vi "Calibration-NormalizeData.vi"(8 "error in (no error)":errorcluster, 11 "Calibration-RunTest in":refnum<class "Calibration-RunTest.lvclass">) -> (0 "error out":errorcluster, 3 "Calibration-RunTest out":refnum<class "Calibration-RunTest.lvclass">)   [LabVIEW 2013, in "Calibration-RunTest.lvclass"]
uses:
  Calibration-RunTest.lvclass
  Calibration-RunTest.lvclass/Calibration-RunTest.ctl
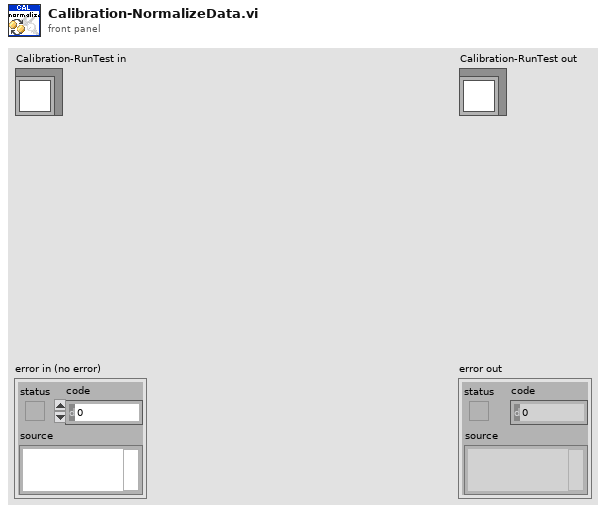
[diagram p1: front panel]
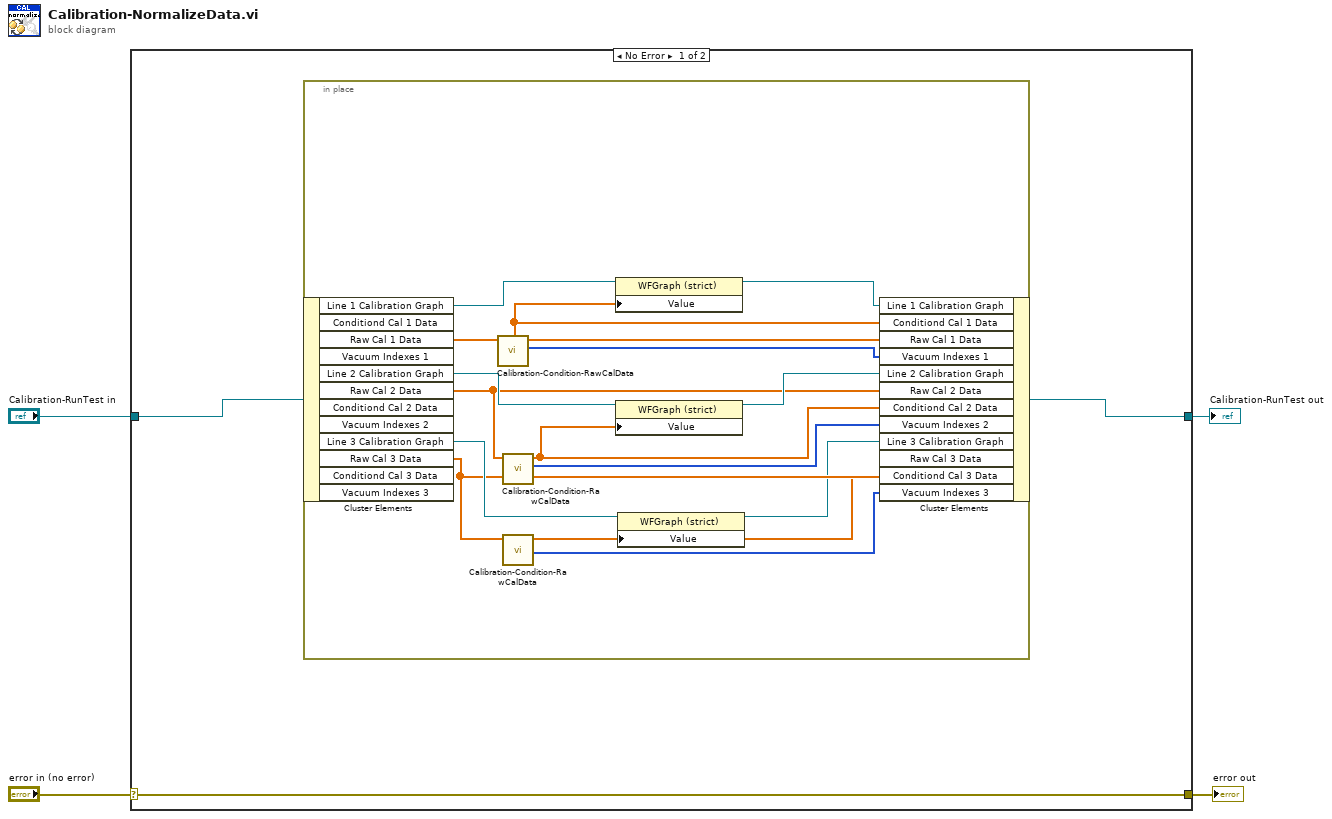
[diagram p0: block diagram]
diagram:
  n1 = case shown="No Error" "error in (no error)" {
    selector: "error in (no error)" -> [w5 w24]
    tunnel: [w5 w24] -> w3
    tunnel: [w6 w23] -> w1
    tunnel: "Calibration-RunTest in" -> [w7 w23]
    frame No Error {
      n2 = in-place {
        n3 = in-place-cluster #1(w7) -> ("Line 1 Calibration Graph"=w9:refnum<vi>, "Raw Cal 1 Data"=w22:dbl[], "Line 2 Calibration Graph"=w19:refnum<vi>, "Raw Cal 2 Data"=w17:dbl[], "Line 3 Calibration Graph"=w14:refnum<vi>, "Raw Cal 3 Data"=w13:dbl[])  [unwired: 6 out]
        n4 = call "Calibration-Condition-RawCalData.vi"("Raw Cal 1 Data In"=w22) -> ("sorted array of indexes"=w20:i32[], "conditioned Output Array"=w21:dbl[])  [unwired: 9 in]
        n5 = call "Calibration-Condition-RawCalData.vi"("Raw Cal 1 Data In"=w17) -> ("sorted array of indexes"=w15:i32[], "conditioned Output Array"=w16:dbl[])  [unwired: 9 in]
        n6 = call "Calibration-Condition-RawCalData.vi"("Raw Cal 1 Data In"=w13) -> ("sorted array of indexes"=w10:i32[], "conditioned Output Array"=w11:dbl[])  [unwired: 9 in]
        n7 = property class="WFGraph (strict)"(reference=w9, "Value"=w21) -> (reference out=w8:refnum<vi>)  [unwired: 1 in, 1 out]
        n8 = property class="WFGraph (strict)"(reference=w19, "Value"=w16) -> (reference out=w18:refnum<vi>)  [unwired: 1 in, 1 out]
        n9 = property class="WFGraph (strict)"(reference=w14, "Value"=w11) -> (reference out=w12:refnum<vi>)  [unwired: 1 in, 1 out]
        n10 = in-place-cluster #1("Line 1 Calibration Graph"=w8, "Conditiond Cal 1 Data"=w21, "Raw Cal 1 Data"=w22, "Vacuum Indexes 1"=w20, "Line 2 Calibration Graph"=w18, "Raw Cal 2 Data"=w17, "Conditiond Cal 2 Data"=w16, "Vacuum Indexes 2"=w15, "Line 3 Calibration Graph"=w12, "Raw Cal 3 Data"=w13, "Conditiond Cal 3 Data"=w11, "Vacuum Indexes 3"=w10) -> (w6:refnum<class "Calibration-RunTest.lvclass">)
      }
    }
    frame Error {
    }
  }
  "error out" <- w3
  "Calibration-RunTest out" <- w1
